vi "HEWH Flow and Temp Adjustment.vi"(0 "MW100":refnum<visa-resource-name>, 1 "FlowReading":dbl, 2 "Flow In":dbl=2.9360496277915633, 3 "K(0.1)":dbl=0.1, 4 "TempReading":dbl, 5 "Error In":errorcluster, 6 "FlowTarget":dbl=3.0, 7 "Temp Target":dbl=58.0, 9 "Temp In":dbl=2.9360496277915633, 10 "Semiphore":T1, 11 "Elapsed Time (sec)":dbl format="%.2f", 13 "Flow Adjust Time (3s)":dbl=1.5) -> (15 "Flow Out":dbl, 18 "Temp Out":dbl, 19 "Error Out":errorcluster)   [LabVIEW 2012]
uses:
  TestedFlowratesScenarios.ctl
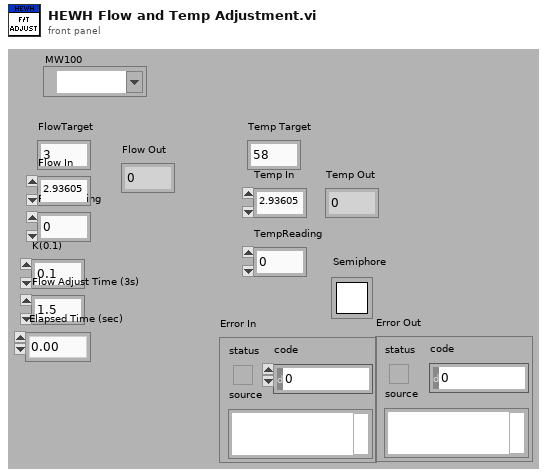
[diagram p1: front panel]
types:
  T1 = typedef "Semaphore RefNum" = refnum<k1>
  T2 = typedef "TestedFlowratesScenarios.ctl" = enum16{"DRK500,Station1", "DRK375,Lab", "SRK500,Station1,5GPM FR", "DRK375,STATION3,1/2\"HOSE", "DRK500,Station1,downspout", "DRK375,Station3,thruEcocute", "DRK375,Station3,purge", "Build2,2B,Purge", "Global, Purge", "Global, Tank"}
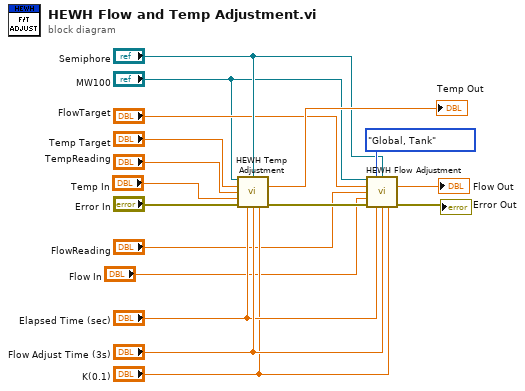
[diagram p0: block diagram]
diagram:
  n1 = call "HEWH Temp Adjustment.vi"("VISA session"="MW100", "Semiphore"="Semiphore", "Degrees Target(58)"="Temp Target", "Degrees reading"="TempReading", "Degrees setting In"="Temp In", "Error In"="Error In", "Elapsed Time (sec)"="Elapsed Time (sec)", "Temp Adjust Time (3s)"="Flow Adjust Time (3s)", "K(0.1)"="K(0.1)") -> ("Degree setting Out"=→"Temp Out":dbl, "Error Out"=w15:errorcluster)  [unwired: 4 in, 1 out]
  n2 = call "HEWH Flow Adjustment.vi"("VISA session"="MW100", "Configuration"=TestedFlowratesScenarios."Global, Tank" ("Draw Test Condition"), "Semiphore"="Semiphore", "GPM Target(3)"="FlowTarget", "GPM reading"="FlowReading", "Flow rate setting In"="Flow In", "Error In"=w15, "Elapsed Time (sec)"="Elapsed Time (sec)", "Flow Adjust Time (3s)"="Flow Adjust Time (3s)", "K(0.1)"="K(0.1)") -> ("Flow rate setting Out"=→"Flow Out":dbl, "Error Out"=→"Error Out":errorcluster)  [unwired: 3 in, 1 out]
